vi "Main.vi"(11 "Module Admin":refnum<class "Delacor_lib_QMH_Module Admin.lvclass">) -> ()   [LabVIEW 2020, in "Acquisition .lvlib"]
doc: "This template is based off of the Queued Message Handler design pattern and the Queued Message Handler project template that ships with LabVIEW.\n\nThe main difference is that the queue is private to this module and communication between modules is performed via Broadcast and Request events.\n\nRequest events are wrapped in public API methods and are handled in the Event Handling Loop (EHL) of this VI. Any module can register for Broadcast events sent by this module. The EHL generates messages based on user interface actions.\n\nThe Message Handling Loop (MHL) processes messages generated by the EHL, or by other messages. The messages are string values, so new messages can be added easily to the Message Cases case structure in the MHL. Each message cluster can also provide an optional value for Message Data, which is a variant that can be converted to whatever message-specific data is required.\n_____\nBased on Delacor QMH Project Template 6.0.0.89."
uses:
  Acquisition .lvlib
  <vilib>/Delacor/Delacor QMH/Libraries/Module Admin_class/Delacor_lib_QMH_Module Admin.lvclass
  Module Data--cluster.ctl
  Stop Argument--cluster.ctl
  <vilib>/Delacor/Delacor QMH/Libraries/Message Queue_class/Delacor_lib_QMH_Message Queue.lvclass/Delacor_lib_QMH_Message Queue.ctl
  <vilib>/Delacor/Delacor QMH/Libraries/Module Admin_class/Delacor_lib_QMH_Module Admin.lvclass/Delacor_lib_QMH_Module Admin.ctl
  Start Analog AQ Argument--cluster.ctl
  Start Digital AQ Argument--cluster.ctl
  Stop AQ Argument--cluster.ctl
  <vilib>/Utility/miscctls.llb/LVPointTypeDef.ctl
  <vilib>/DAQmx/read.llb/DAQmx Read (Digital 1D U8 NChan 1Samp).vi
  <vilib>/DAQmx/read.llb/DAQmx Read (Analog 1D Wfm NChan NSamp).vi
  <vilib>/Delacor/Delacor QMH/Libraries/Message Queue_class/Delacor_lib_QMH_Enqueue Message (Single).vi
  <vilib>/Delacor/Delacor QMH/Libraries/Module Admin_class/Delacor_lib_QMH_Get External Launch.vi
  <vilib>/DAQmx/miscellaneous.llb/DAQmx Fill In Error Info.vi
  <vilib>/Utility/error.llb/Error Cluster From Error Code.vi
  <vilib>/ErrorRing/Error Ring.xnode
  <vilib>/Delacor/Delacor QMH/Libraries/Message Queue_class/Delacor_lib_QMH_Message Queue.lvclass
panel:
  out "error out":errorcluster
  out "Status":string
types:
  T1 = typedef "Acquisition .lvlib/Request Events--cluster.ctl" = cluster{"Stop Module":refnum<user-event>, "Show Panel":refnum<user-event>, "Hide Panel":refnum<user-event>, "Get Module Execution Status":refnum<user-event>, "Show Diagram":refnum<user-event>, "WakeUp Analog HL":refnum<user-event>, "WakeUp Digital HL":refnum<user-event>, "Put HL to Sleep":refnum<user-event>, "Start Analog AQ":refnum<user-event>, "Start Digital AQ":refnum<user-event>, "Stop AQ":refnum<user-event>}
  T2 = typedef "Acquisition .lvlib/Module Data--cluster.ctl" = cluster{"Status":string, "Analog Signal":cluster{"DAQ Board Name":tag, "Canales":tag[], "rate":dbl, "number of samples ":i32, "Tiempo":dbl}, "digital Signal":cluster{"DAQ Board Name":tag, "Canales":tag[], "rate":i32, "Tiempo ":dbl}}
  T3 = enum32{"invalid lock state", "Not Locked", "Locked (No Password)", "Password-protected"}
  T4 = typedef "Acquisition .lvlib/Stop Argument--cluster.ctl" = cluster{"Origin":string, "Exit via Stop Module Req?":bool, "Wait for Module to stop?":bool}
  T5 = typedef "Acquisition .lvlib/Start Analog AQ Argument--cluster.ctl" = cluster{"Boolean":bool}
  T6 = typedef "Acquisition .lvlib/Start Digital AQ Argument--cluster.ctl" = cluster{"Boolean":bool}
  T7 = typedef "Acquisition .lvlib/Stop AQ Argument--cluster.ctl" = cluster{"Boolean":bool}
  T8 = typedef "LVPointTypeDef.ctl" = cluster{"Horizontal":i16, "Vertical":i16}
  T9 = enum32{"Invalid", "Standard", "Closed", "Hidden", "Minimized", "Maximized"}
  T10 = cluster{"DAQ Board Name":tag, "Canales":tag[], "rate":dbl, "number of samples ":i32, "Tiempo":dbl}
  T11 = cluster{"DAQ Board Name":tag, "Canales":tag[], "rate":i32, "Tiempo ":dbl}
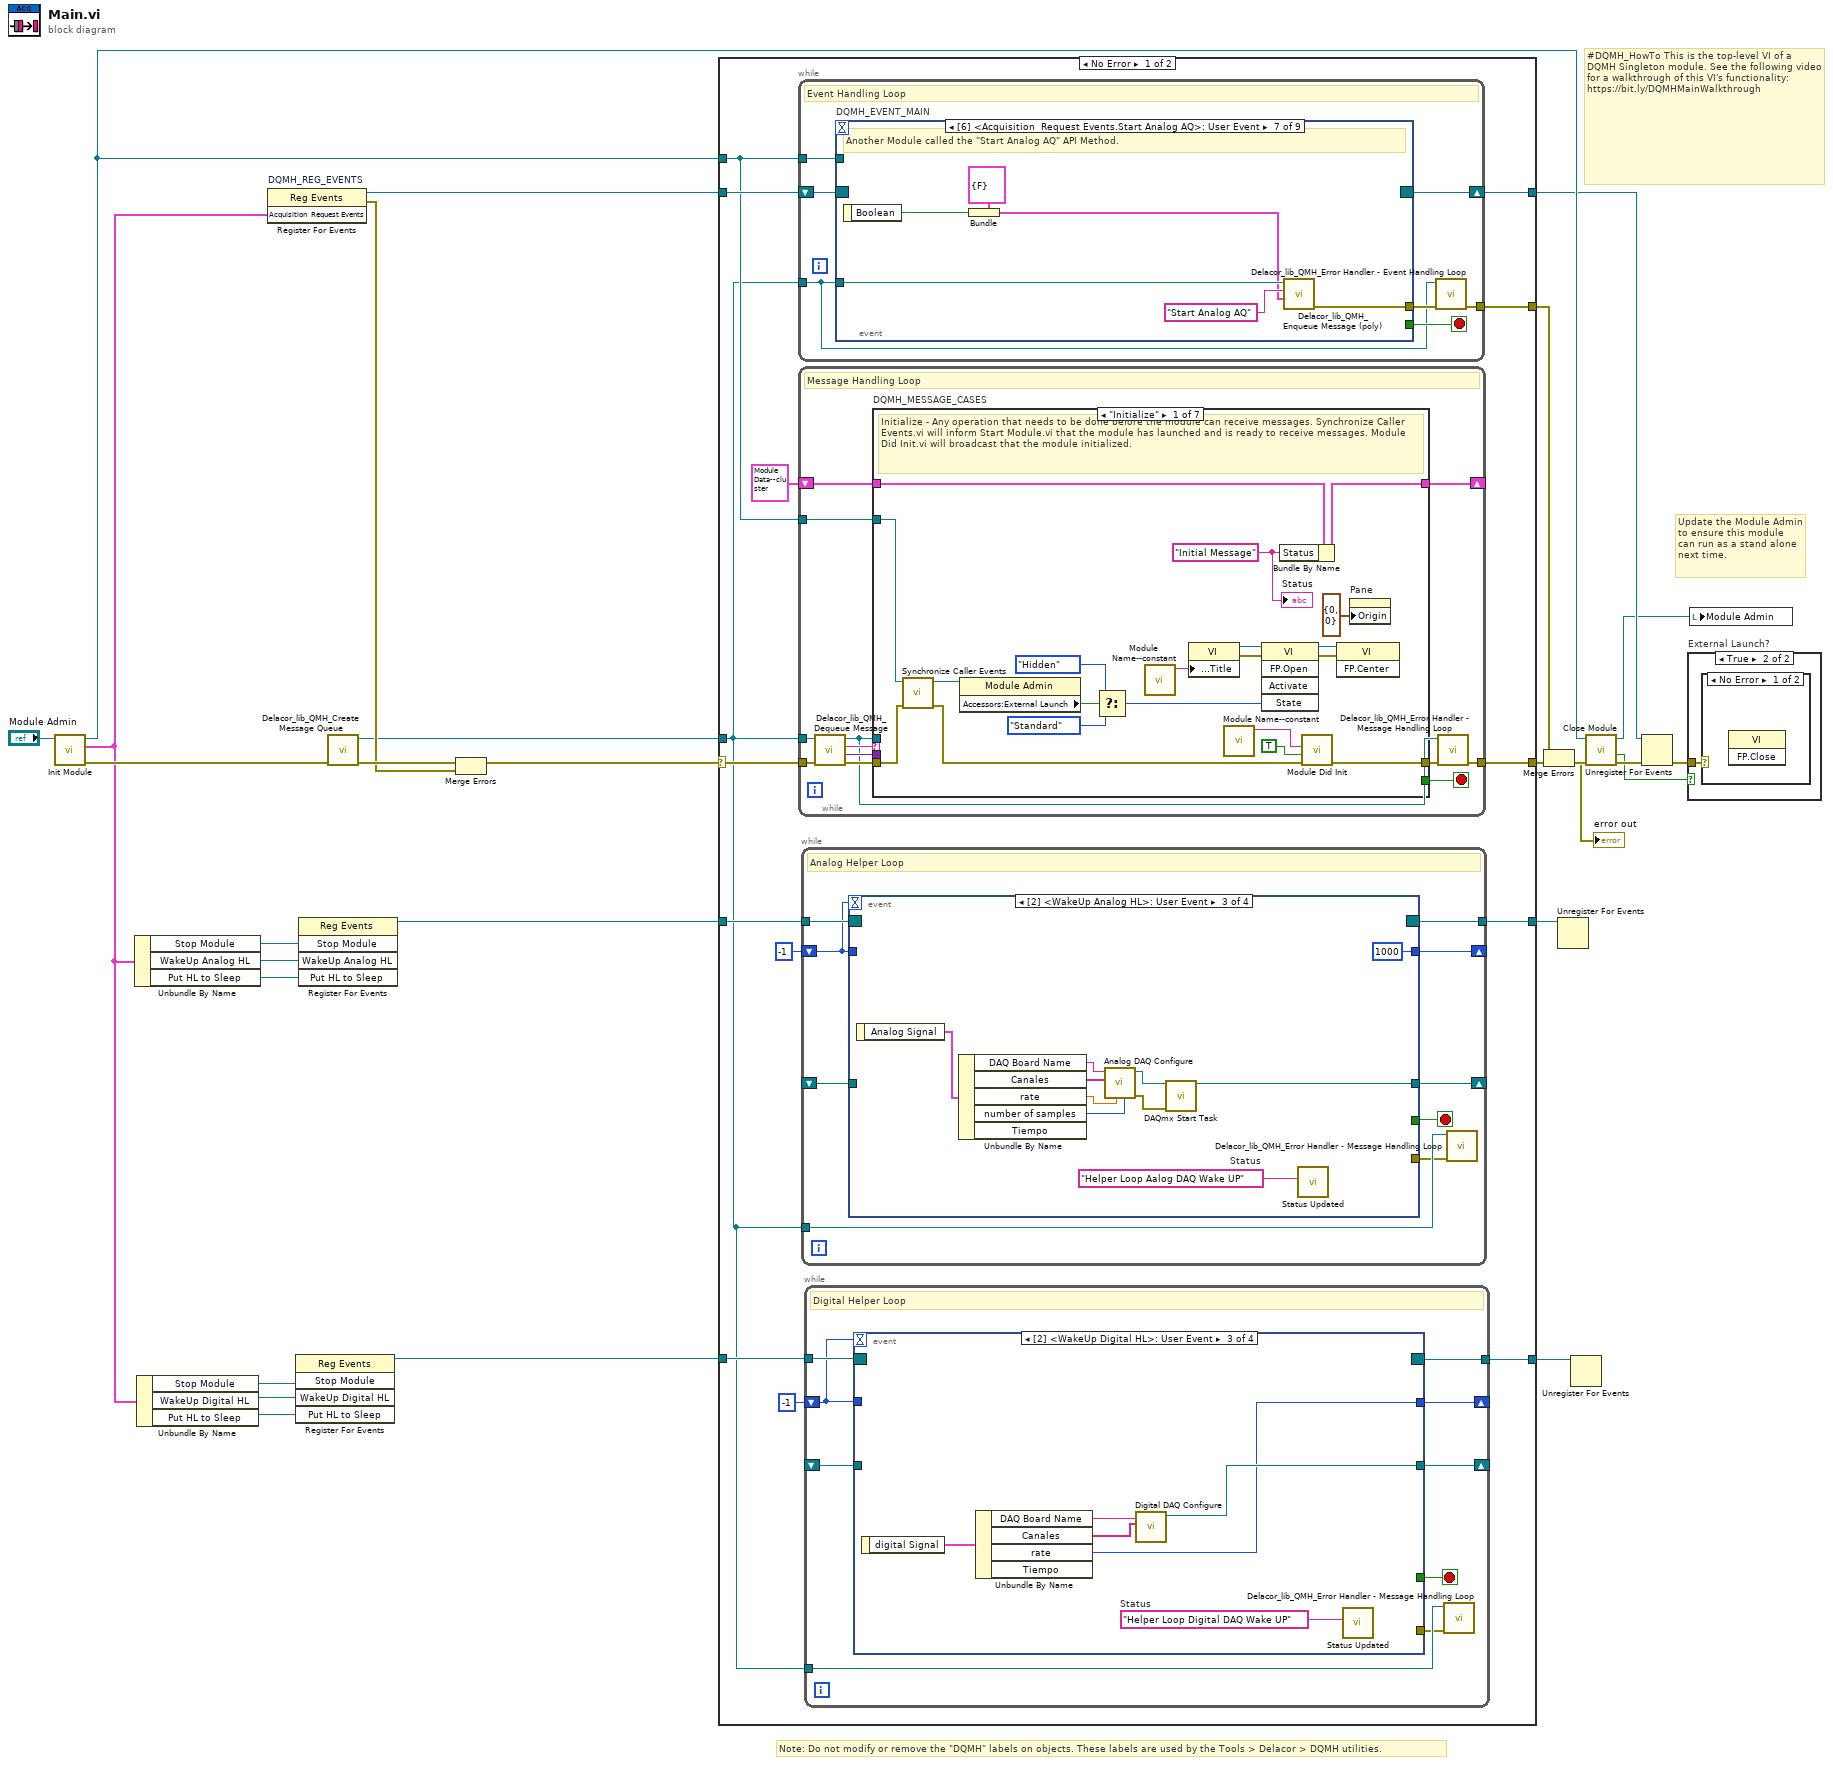
[diagram p0: block diagram]
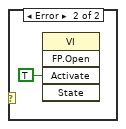
[diagram p3: hidden frame]
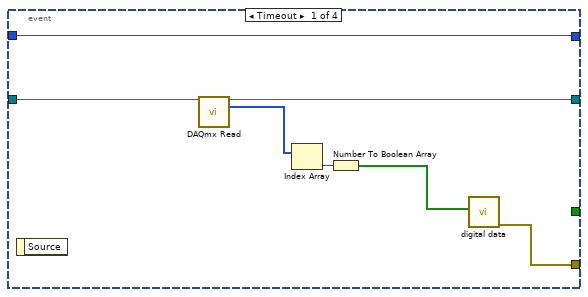
[diagram p4: hidden frame]
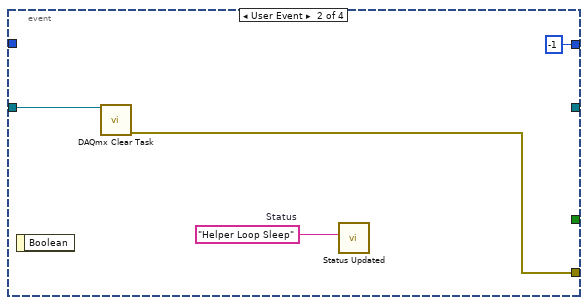
[diagram p5: hidden frame]
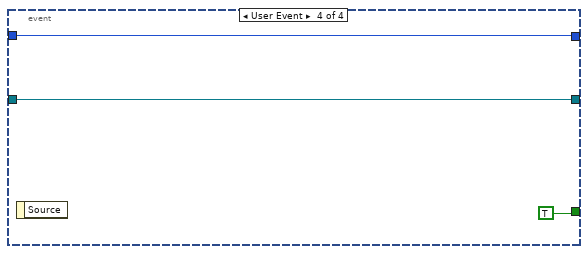
[diagram p6: hidden frame]
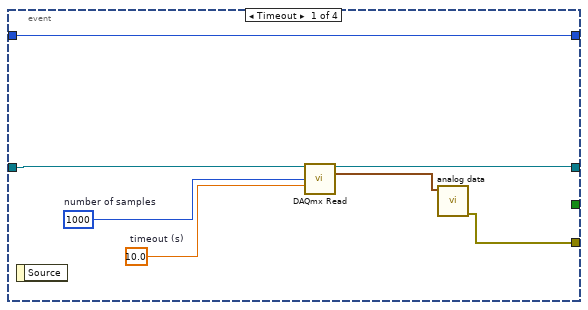
[diagram p7: hidden frame]
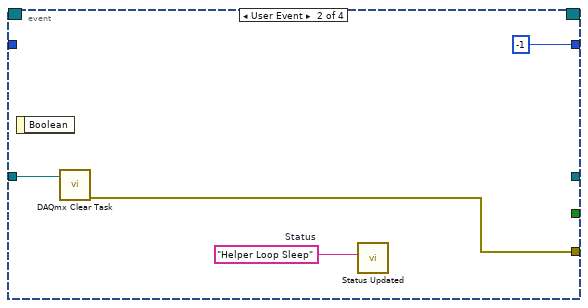
[diagram p8: hidden frame]
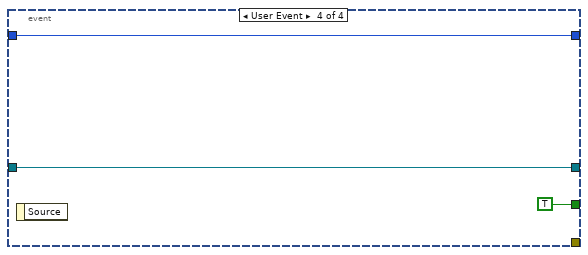
[diagram p9: hidden frame]
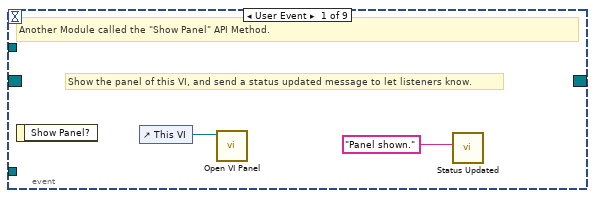
[diagram p10: hidden frame]
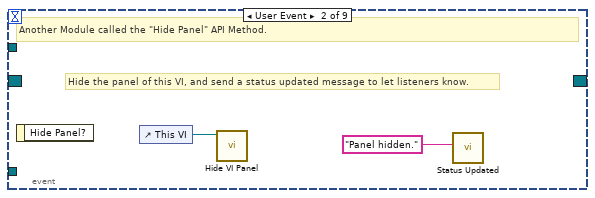
[diagram p11: hidden frame]
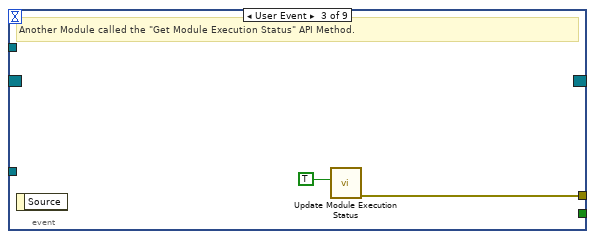
[diagram p12: hidden frame]
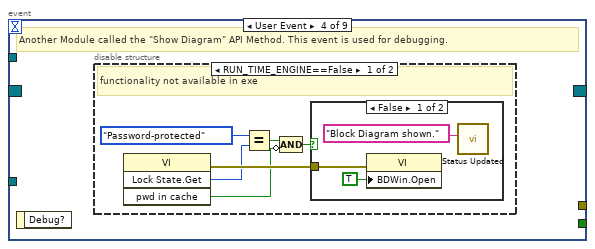
[diagram p13: hidden frame]
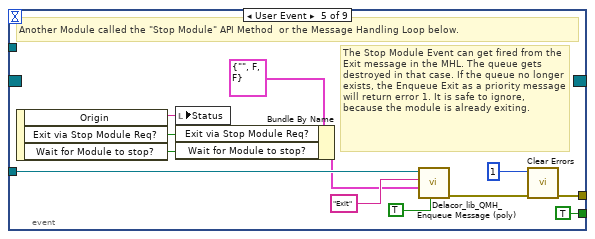
[diagram p16: hidden frame]
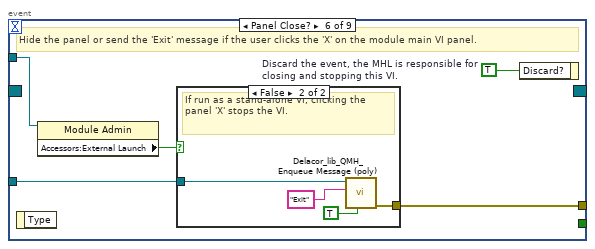
[diagram p17: hidden frame]
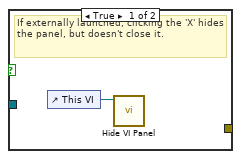
[diagram p18: hidden frame]
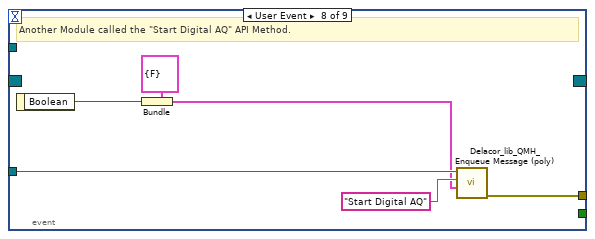
[diagram p19: hidden frame]
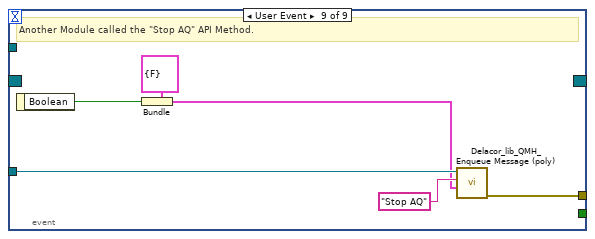
[diagram p20: hidden frame]
diagram:
  # "#DQMH_HowTo This is the top-level VI of a DQMH Singleton module. See the following video for a walkthrough of this VI's functionality: https://bit.ly/DQMHMainWalkthrough"
  # "Note: Do not modify or remove the \"DQMH\" labels on objects. These labels are used by the Tools > Delacor > DQMH utilities."
  # "Update the Module Admin to ensure this module can run as a stand alone next time."
  n1 = call "Init Module.vi"("Singleton Module Admin in"="Module Admin") -> ("error out"=w26:errorcluster, "Acquisition  Request Events"=w8:T1, "Singleton Module Admin out"=w18:refnum<class "Delacor_lib_QMH_Module Admin.lvclass">)  [unwired: 8 in]
  n2 = Unbundle By Name(w8) -> ("Stop Module"=w9:refnum<user-event>, "WakeUp Analog HL"=w10:refnum<user-event>, "Put HL to Sleep"=w11:refnum<user-event>)
  n3 = Unbundle By Name(w8) -> ("Stop Module"=w5:refnum<user-event>, "WakeUp Digital HL"=w6:refnum<user-event>, "Put HL to Sleep"=w7:refnum<user-event>)
  n4 = register-events "DQMH_REG_EVENTS"(w8) -> (reference out=w16:refnum<event-registration>, error out=w19:errorcluster)  [unwired: 2 in]
  n5 = register-events(w5, w6, w7) -> (reference out=w4:refnum<event-registration>)  [unwired: 2 in, 1 out]
  n6 = register-events(w9, w10, w11) -> (reference out=w3:refnum<event-registration>)  [unwired: 2 in, 1 out]
  n7 = call <vilib>:"Delacor_lib_QMH_Create Message Queue.vi"("error in"=w26) -> ("error out"=w21:errorcluster, "Message Queue"=w15:refnum<class "Delacor_lib_QMH_Message Queue.lvclass">)  [unwired: 9 in]
  n8 = Merge Errors(w21, w19) -> (w20:errorcluster)
  n9 = case shown="No Error" w20 {
    selector: w20 -> [w39 w273]
    tunnel: [w41 w272] -> w27
    tunnel: [w38 w278] -> w17
    tunnel: w16 -> [w36 w278]
    tunnel: w15 -> [w30 w271]
    tunnel: [w40 _] -> w24
    tunnel: w18 -> [w35 w274]
    tunnel: w4 -> [w34 w270]
    tunnel: w3 -> [w33 w269]
    tunnel: [w32 w270] -> w2
    tunnel: [w31 w269] -> w1
    frame No Error {
      n10 = while {
        tunnel: w30 -> [w104]
        shift-right: [w107] -> w38
        shift-left: w36 -> [w108]
        tunnel: [w109] -> w40
        tunnel: w35 -> [w105]
        stop <- w106 stop-if-true
        # "Event Handling Loop"
        n11 = event "DQMH_EVENT_MAIN" shown="[6] <Acquisition  Request Events.Start Analog AQ>: User Event" {
          selector: w108 -> [_ _ _ _ _ _ _ _ _]
          dyn-events: [_ _ _ _ _ _ _ _ _] -> w107
          timeout: _ -> [_ _ _ _ _ _ _ _ _]
          tunnel: [_ _ _ _ TRUE ("Discard?") _ _ _ _] -> w106
          tunnel: w104 -> [_ _ _ _ w133 w140 w153 w159 w165]
          tunnel: [_ _ w116 _ w136 w142 w148 w154 w160] -> w110
          tunnel: w105 -> [_ _ _ _ _ w139 _ _ _]
          event User Event {
            # "Show the panel of this VI, and send a status updated message to let listeners know."
            # "Another Module called the \"Show Panel\" API Method."
            n12 = event-data() -> ()  [unwired: 1 in, 1 out]
            n13 = control-ref of="This VI"() -> (w112:refnum<vi>)
            n14 = call "Open VI Panel.vi"("VI"=w112) -> ()  [unwired: 10 in, 1 out]
            n15 = call "Status Updated.vi"("Status"="Panel shown." ("format string")) -> ()  [unwired: 10 in, 1 out]
          }
          event User Event {
            # "Hide the panel of this VI, and send a status updated message to let listeners know."
            # "Another Module called the \"Hide Panel\" API Method."
            n16 = event-data() -> ()  [unwired: 1 in, 1 out]
            n17 = control-ref of="This VI"() -> (w114:refnum<vi>)
            n18 = call "Hide VI Panel.vi"("VI"=w114) -> ()  [unwired: 10 in, 1 out]
            n19 = call "Status Updated.vi"("Status"="Panel hidden." ("format string")) -> ()  [unwired: 10 in, 1 out]
          }
          event User Event {
            # "Another Module called the \"Get Module Execution Status\" API Method."
            n20 = event-data() -> ()  [unwired: 1 in, 1 out]
            n21 = call "Update Module Execution Status.vi"("Running?"=TRUE) -> ("error out"=w116:errorcluster)  [unwired: 10 in]
          }
          event User Event {
            # "Another Module called the \"Show Diagram\" API Method. This event is used for debugging."
            n22 = event-data() -> ()  [unwired: 1 in, 1 out]
            n23 = disable-structure shown="RUN_TIME_ENGINE==False" {
              frame condition #0 (active) {
                # "functionality not available in exe"
                n24 = invoke class="VI" method="Lock State.Get"() -> (error out=w122:errorcluster, "Get Lock State"=w121:T3, "pwd in cache"=w118:bool)  [unwired: 4 in, 1 out]
                n25 = Equal?(x=T3."Password-protected", y=w121) -> (x = y?=w119:bool)
                n26 = Compound Arithmetic op=AND(w119, invert w118) -> (w117:bool)
                n27 = case shown="False" w117 {
                  tunnel: w122 -> [w125 _]
                  frame False {
                    n28 = property class="VI"(error in=w125, "BDWin.Open"=TRUE ("Block Diagram Window:Open")) -> ()  [unwired: 1 in, 2 out]
                    n29 = call "Status Updated.vi"("Status"="Block Diagram shown." ("format string")) -> ()  [unwired: 10 in, 1 out]
                  }
                  frame True {
                    # "Password-protected VI, and the password is not in the cache. Do not show the diagram."
                  }
                }
              }
              frame condition #1 {
              }
            }
          }
          event User Event {
            # "The Stop Module Event can get fired from the Exit message in the MHL. The queue gets destroyed in that case. If the queue no longer exists, the Enqueue Exit as a priority message will return error 1. It is safe to ignore, because the module is already exiting."
            # "Another Module called the \"Stop Module\" API Method  or the Message Handling Loop below."
            n30 = event-data() -> ("Origin"=w132:string, "Exit via Stop Module Req?"=w128:bool, "Wait for Module to stop?"=w127:bool)  [unwired: 1 in]
            n31 = local write "Status"(w132) -> ()
            n32 = Bundle By Name(cluster=T4 {"Origin"="", "Exit via Stop Module Req?"=FALSE, "Wait for Module to stop?"=FALSE} ("Stop Argument"), "Exit via Stop Module Req?"=w128, "Wait for Module to stop?"=w127) -> (w126:T4)
            n33 = call-poly <vilib>:"Delacor_lib_QMH_Enqueue Message (poly).vi"("Priority Message? (F)"=TRUE, "Message Data"=w126, "Message"="Exit", "Message Queue in"=w133) -> ("error out"=w137:errorcluster)  [unwired: 6 in, 1 out]
            n34 = call <vilib>:"Clear Errors.vi"("error in (no error)"=w137, "specific error code to clear (0: all)"=1) -> ("error out"=w136:errorcluster)  [unwired: 4 in, 1 out]
          }
          event Panel Close? {
            w141 = TRUE  # Discard the event, the MHL is responsible for closing and stopping this VI.
            # "Hide the panel or send the 'Exit' message if the user clicks the 'X' on the module main VI panel."
            n35 = event-data() -> ()  [unwired: 1 in, 1 out]
            n36 = property class="Module Admin"(reference=w139) -> ("Accessors:External Launch"=w138:bool)  [unwired: 1 in, 2 out]
            n37 = case shown="False" w138 {
              tunnel: w140 -> [_ w146]
              tunnel: [_ w147] -> w142
              frame True {
                # "If externally launched, clicking the 'X' hides the panel, but doesn't close it."
                n38 = control-ref of="This VI"() -> (w143:refnum<vi>)
                n39 = call "Hide VI Panel.vi"("VI"=w143) -> ()  [unwired: 10 in, 1 out]
              }
              frame False {
                # "If run as a stand-alone VI, clicking the panel 'X' stops the VI."
                n40 = call-poly <vilib>:"Delacor_lib_QMH_Enqueue Message (poly).vi"("Priority Message? (F)"=TRUE, "Message"="Exit", "Message Queue in"=w146) -> ("error out"=w147:errorcluster)  [unwired: 7 in, 1 out]
              }
            }
            n41 = event-data("Discard?"=w141) -> ()  [unwired: 1 in, 1 out]
          }
          event User Event {
            # "Another Module called the \"Start Analog AQ\" API Method."
            n42 = event-data() -> ("Boolean"=w149:bool)  [unwired: 1 in]
            n43 = Bundle(cluster=T5 {"Boolean"=FALSE} ("Start Analog AQ Argument"), "Boolean"=w149) -> (w150:T5)
            n44 = call-poly <vilib>:"Delacor_lib_QMH_Enqueue Message (poly).vi"("Message Data"=w150, "Message"="Start Analog AQ", "Message Queue in"=w153) -> ("error out"=w148:errorcluster)  [unwired: 7 in, 1 out]
          }
          event User Event {
            # "Another Module called the \"Start Digital AQ\" API Method."
            n45 = event-data() -> ("Boolean"=w155:bool)  [unwired: 1 in]
            n46 = Bundle(cluster=T6 {"Boolean"=FALSE} ("Start Digital AQ Argument"), "Boolean"=w155) -> (w156:T6)
            n47 = call-poly <vilib>:"Delacor_lib_QMH_Enqueue Message (poly).vi"("Message Data"=w156, "Message"="Start Digital AQ", "Message Queue in"=w159) -> ("error out"=w154:errorcluster)  [unwired: 7 in, 1 out]
          }
          event User Event {
            # "Another Module called the \"Stop AQ\" API Method."
            n48 = event-data() -> ("Boolean"=w161:bool)  [unwired: 1 in]
            n49 = Bundle(cluster=T7 {"Boolean"=FALSE} ("Stop AQ Argument"), "Boolean"=w161) -> (w162:T7)
            n50 = call-poly <vilib>:"Delacor_lib_QMH_Enqueue Message (poly).vi"("Message Data"=w162, "Message"="Stop AQ", "Message Queue in"=w165) -> ("error out"=w160:errorcluster)  [unwired: 7 in, 1 out]
          }
        }
        n51 = call-dynamic "Delacor_lib_QMH_Error Handler - Event Handling Loop.vi"("error in"=w110, "Message Queue in"=w104) -> ("dup error in"=w109:errorcluster)  [unwired: 8 in, 1 out]
      }
      n52 = while {
        tunnel: w30 -> [w168]
        shift-right: [w172] -> _
        shift-left: T2 {"Status"="", "Analog Signal"={"DAQ Board Name"="", "Canales"=[], "rate"=0.0, "number of samples "=0, "Tiempo"=0.0}, "digital Signal"={"DAQ Board Name"="", "Canales"=[], "rate"=1000, "Tiempo "=1000.0}} ("Data Cluster") -> [w173]
        tunnel: w39 -> [w176]
        tunnel: [w174] -> w41
        tunnel: w35 -> [w166]
        stop <- w171 stop-if-true
        # "Message Handling Loop"
        n53 = call-dynamic "Delacor_lib_QMH_Dequeue Message.vi"("error in"=w176, "Message Queue in"=w168) -> ("error out"=w175:errorcluster, "Message Data"=w169:variant, "Message"=w170:string, "Message Queue out"=w167:refnum<class "Delacor_lib_QMH_Message Queue.lvclass">)  [unwired: 6 in]
        n54 = case "DQMH_MESSAGE_CASES" shown="\"Initialize\"" w170 {
          selector: w170 -> [_ _ _ w230 _ _ _]
          tunnel: w167 -> [_ w200 w222 _ _ _ _]
          tunnel: w175 -> [w195 w207 w228 w232 w251 w260 w268]
          tunnel: [w193 w203 w225 w233 w245 w254 w262] -> w177
          tunnel: w173 -> [w184 w202 w221 w231 w246 w255 w267]
          tunnel: [w183 w202 w221 w231 w246 w255 w267] -> w172
          tunnel: [_ _ w220 _ _ _ _] -> w171
          tunnel: w169 -> [_ w201 w219 _ w249 w258 w265]
          tunnel: w166 -> [w185 w199 w214 _ _ _ _]
          frame "Initialize" {
            w179 = "Initial Message" ("Initial Message")
            # "Initialize - Any operation that needs to be done before the module can receive messages. Synchronize Caller Events.vi will inform Start Module.vi that the module has launched and is ready to receive messages. Module Did Init.vi will broadcast that the module initialized."
            n55 = call "Synchronize Caller Events.vi"("error in (no error)"=w195, "Singleton Module Admin in"=w185) -> ("error out"=w194:errorcluster, "Singleton Module Admin out"=w180:refnum<class "Delacor_lib_QMH_Module Admin.lvclass">)  [unwired: 8 in]
            n56 = property class="Module Admin"(reference=w180) -> ("Accessors:External Launch"=w189:bool)  [unwired: 1 in, 2 out]
            n57 = Select(t=T9."Hidden" ("State"), s=w189, f=T9."Standard" ("State")) -> (s? t:f=w186:T9)
            n58 = call "Module Name--constant.vi"() -> ("Module Name"=w192:string)  [unwired: 11 in]
            n59 = property class="VI"("Front Panel.Title"=w192) -> (reference out=w191:refnum<vi>, error out=w197:errorcluster)  [unwired: 2 in]
            n60 = call "Module Name--constant.vi"() -> ("Module Name"=w181:string)  [unwired: 11 in]
            n61 = invoke class="VI" method="FP.Open"(reference=w191, error in=w197, "State"=w186) -> (reference out=w190:refnum<vi>, error out=w196:errorcluster)  [unwired: 2 in, 3 out]
            n62 = Bundle By Name(cluster=w184, "Status"=w179) -> (w183:T2)
            n63 = call "Module Did Init.vi"("error in (no error)"=w194, "Initialized?"=TRUE, "Origin"=w181) -> ("error out"=w193:errorcluster)  [unwired: 8 in]
            n64 = invoke class="VI" method="FP.Center"(reference=w190, error in=w196) -> ()  [unwired: 1 in, 3 out]
            n65 = property on="Pane" class="Pane"("Origin"=T8 {"Horizontal"=0, "Vertical"=0}) -> ()  [unwired: 2 in, 2 out]
            "Status" <- w179
          }
          frame "Error" {
            # "#CodeRecommended - If you ever change the name of this \"Error\" message, you'll need to update the name in the Check Loop Error.vi as well."
            # "#CodeRecommended - If the module is running in standalone mode (External Launch = FALSE), this code will pop up an error dialog and call the 'Exit' message if an error occurs. Add more fine-grained error handling here."
            # "Error - Check the error message data and respond accordingly. This message is sent by the \"Error Handler\" VIs at the end of each loop in this application."
            n66 = property class="Module Admin"(reference=w199) -> ("Accessors:External Launch"=w198:bool)  [unwired: 1 in, 2 out]
            n67 = Variant To Data(error in=w207, type=errorcluster {"status"=FALSE, "code"=0, "source"=""} ("error constant"), Variant=w201) -> (data=w208:errorcluster, error out=w205:errorcluster)
            n68 = call "Error Reported.vi"("Error"=w208) -> ()  [unwired: 10 in, 1 out]
            n69 = case shown="False" w198 {
              tunnel: [w213 _] -> w204
              tunnel: w200 -> [w211 _]
              tunnel: w208 -> [w212 _]
              frame False {
                # "If the module is running standalone, then pop up an error dialog and call the \"Exit\" message."
                n70 = call <vilib>:"Simple Error Handler.vi"("error in (no error)"=w212) -> ()  [unwired: 4 in, 5 out]
                n71 = call-poly <vilib>:"Delacor_lib_QMH_Enqueue Message (poly).vi"("Priority Message? (F)"=TRUE, "Message"="Exit", "Message Queue in"=w211) -> ("error out"=w213:errorcluster)  [unwired: 7 in, 1 out]
              }
              frame True {
                # "If the module was launched externally, calling the Error Reported broadcast VI is the only action performed by the \"Error\" message. The module's caller can then process the error appropriately."
              }
            }
            n72 = Merge Errors(w205, w204) -> (w203:errorcluster)
            n73 = local write "error out"(w203) -> ()
          }
          frame "Exit" {
            w218 = 91  # 91: not all Exit messages will have an argument
            w220 = TRUE  # Stop the VI
            # "Release the message queue reference"
            # "#CodeNeeded - Add any required cleanup code here"
            # "Exit - Exit the application."
            n74 = Variant To Data(error in=w228, type=T4 {"Origin"="", "Exit via Stop Module Req?"=FALSE, "Wait for Module to stop?"=FALSE} ("Stop Argument"), Variant=w219) -> (data=w216:T4, error out=w224:errorcluster)
            n75 = call <vilib>:"Clear Errors.vi"("error in (no error)"=w224, "specific error code to clear (0: all)"=w218) -> ("error out"=w227:errorcluster)  [unwired: 4 in, 1 out]
            n76 = control-ref of="This VI"() -> (w215:refnum<vi>)
            n77 = call-dynamic "Delacor_lib_QMH_Release Message Queue.vi"("error in"=w227, "Message Queue"=w222) -> ("error out"=w226:errorcluster)  [unwired: 9 in]
            n78 = call "Handle Exit.vi"("Stop Argument"=w216, "Admin in"=w214, "VI reference"=w215) -> ("error out"=w223:errorcluster)  [unwired: 7 in, 1 out]
            n79 = Merge Errors(w226, w223) -> (w225:errorcluster)
          }
          frame Default {
            # "'Default' case only runs if there is a message that isn't defined in any of the other cases.  Output a programming error."
            n80 = call "Module Name--constant.vi"() -> ("Module Name"=w229:string)  [unwired: 11 in]
            n81 = xnode "Error Ring"("parameter 0"=w230, "parameter 1"=w229) -> ("error out"=w234:errorcluster)
            n82 = Merge Errors(w232, w234) -> (w233:errorcluster)
          }
          frame "Start Analog AQ" {
            # "#wakeUp_analog__HL"
            # "start the analog acquisition"
            n83 = Variant To Data(error in=w251, type=T5 {"Boolean"=FALSE} ("Start Analog AQ Argument"), Variant=w249) -> (data=w247:T5, error out=w250:errorcluster)
            n84 = Unbundle By Name(w247) -> ()  [unwired: 1 out]
            n85 = Unbundle By Name(w246) -> ("Analog Signal"=w243:T10)
            n86 = call "WakeUp Analog HL.vi"("Analog Signal"=w243) -> ("error out"=w244:errorcluster)  [unwired: 10 in]
            n87 = Merge Errors(w244, w250) -> (w245:errorcluster)
          }
          frame "Start Digital AQ" {
            # "#wakeUp_digital__HL"
            # "Start to acquire digital data"
            n88 = Variant To Data(error in=w260, type=T6 {"Boolean"=FALSE} ("Start Digital AQ Argument"), Variant=w258) -> (data=w256:T6, error out=w259:errorcluster)
            n89 = Unbundle By Name(w256) -> ()  [unwired: 1 out]
            n90 = Unbundle By Name(w255) -> ("digital Signal"=w252:T11)
            n91 = call "WakeUp Digital HL.vi"("digital Signal"=w252) -> ("error out"=w253:errorcluster)  [unwired: 10 in]
            n92 = Merge Errors(w253, w259) -> (w254:errorcluster)
          }
          frame "Stop AQ" {
            # "stop to acquire data"
            n93 = Variant To Data(error in=w268, type=T7 {"Boolean"=FALSE} ("Stop AQ Argument"), Variant=w265) -> (data=w263:T7, error out=w266:errorcluster)
            n94 = Unbundle By Name(w263) -> ()  [unwired: 1 out]
            n95 = call "Put HL to Sleep.vi"() -> ("error out"=w261:errorcluster)  [unwired: 11 in]
            n96 = Merge Errors(w261, w266) -> (w262:errorcluster)
          }
        }
        n97 = call-dynamic "Delacor_lib_QMH_Error Handler - Message Handling Loop.vi"("error in"=w177, "Message Queue in"=w167) -> ("dup error in"=w174:errorcluster)  [unwired: 8 in, 1 out]
      }
      n98 = while {
        tunnel: w33 -> [w79]
        tunnel: [w77] -> w31
        tunnel: w30 -> [w76]
        shift-right: [w75] -> _
        shift-left: _ -> [w74]
        shift-right: [w73] -> _
        shift-left: -1 -> [w72]
        stop <- w78 stop-if-true
        # "Analog Helper Loop"
        n99 = event shown="[2] <WakeUp Analog HL>: User Event" {
          selector: w79 -> [_ _ _ _]
          dyn-events: [_ _ _ _] -> w77
          timeout: w72 -> [_ _ _ _]
          tunnel: [_ _ _ TRUE] -> w78
          tunnel: [w82 _ w96 w101] -> w75
          tunnel: w74 -> [w83 w89 _ w101]
          tunnel: [w86 -1 1000 w102] -> w73
          tunnel: w72 -> [w86 _ _ w102]
          tunnel: [w81 w87 _ _] -> w71
          event Timeout {
            w84 = 10.0  # timeout (s)
            w85 = 1000  # number of samples
            n100 = event-data() -> ()  [unwired: 1 in, 1 out]
            n101 = call-poly <vilib>:"DAQmx Read.vi"("task/channels in"=w83, "number of samples per channel"=w85, "timeout"=w84) -> ("task out"=w82:refnum<k21>, "data"=w80:waveform(dbl)[])  [unwired: 10 in, 1 out]
            n102 = call "analog data.vi"("data"=w80) -> ("error out"=w81:errorcluster)  [unwired: 10 in]
          }
          event User Event {
            w90 = "Helper Loop Sleep"  # Status
            n103 = event-data() -> ()  [unwired: 1 in, 1 out]
            n104 = call <vilib>:"DAQmx Clear Task.vi"("task in"=w89) -> ("error out"=w87:errorcluster)  [unwired: 14 in]
            n105 = call "Status Updated.vi"("Status"=w90) -> ()  [unwired: 10 in, 1 out]
          }
          event User Event {
            w97 = "Helper Loop Aalog DAQ Wake UP"  # Status
            n106 = event-data() -> ("Analog Signal"=w100:T10)  [unwired: 1 in]
            n107 = Unbundle By Name(w100) -> ("DAQ Board Name"=w94:tag, "Canales"=w93:tag[], "rate"=w92:dbl, "number of samples"=w91:i32)  [unwired: 1 out]
            n108 = call "Analog DAQ Configure.vi"("number of samples"=w91, "rate"=w92, "Canales"=w93, "DAQ Board Name"=w94) -> ("error out"=w99:errorcluster, "task out"=w98:refnum<k21>)  [unwired: 6 in]
            n109 = call <vilib>:"DAQmx Start Task.vi"("task/channels in"=w98, "error in"=w99) -> ("task out"=w96:refnum<k21>)  [unwired: 12 in, 1 out]
            n110 = call "Status Updated.vi"("Status"=w97) -> ()  [unwired: 10 in, 1 out]
          }
          event User Event {
            n111 = event-data() -> ()  [unwired: 1 in, 1 out]
          }
        }
        n112 = call-dynamic "Delacor_lib_QMH_Error Handler - Message Handling Loop.vi"("error in"=w71, "Message Queue in"=w76) -> ()  [unwired: 8 in, 2 out]
      }
      n113 = while {
        tunnel: w34 -> [w50]
        tunnel: [w48] -> w32
        tunnel: w30 -> [w47]
        shift-right: [w46] -> _
        shift-left: _ -> [w45]
        shift-right: [w44] -> _
        shift-left: -1 -> [w43]
        stop <- w49 stop-if-true
        # "Digital Helper Loop"
        n114 = event shown="[2] <WakeUp Digital HL>: User Event" {
          selector: w50 -> [_ _ _ _]
          dyn-events: [_ _ _ _] -> w48
          timeout: w43 -> [_ _ _ _]
          tunnel: [_ _ _ TRUE] -> w49
          tunnel: [w55 _ w66 w68] -> w46
          tunnel: w45 -> [w56 w60 _ w68]
          tunnel: [w57 -1 w64 w69] -> w44
          tunnel: w43 -> [w57 _ _ w69]
          tunnel: [w54 w59 _ _] -> w42
          event Timeout {
            n115 = event-data() -> ()  [unwired: 1 in, 1 out]
            n116 = call-poly <vilib>:"DAQmx Read.vi"("task/channels in"=w56) -> ("task out"=w55:refnum<k21>, "data"=w51:u8[])  [unwired: 12 in, 1 out]
            n117 = Index Array(array=w51) -> (element=w52:u8)  [unwired: 1 in]
            n118 = Number To Boolean Array(number=w52) -> (Boolean array=w53:bool[])
            n119 = call "digital data.vi"("Digital Signals"=w53) -> ("error out"=w54:errorcluster)  [unwired: 10 in]
          }
          event User Event {
            w58 = "Helper Loop Sleep"  # Status
            n120 = event-data() -> ()  [unwired: 1 in, 1 out]
            n121 = call <vilib>:"DAQmx Clear Task.vi"("task in"=w60) -> ("error out"=w59:errorcluster)  [unwired: 14 in]
            n122 = call "Status Updated.vi"("Status"=w58) -> ()  [unwired: 10 in, 1 out]
          }
          event User Event {
            w65 = "Helper Loop Digital DAQ Wake UP"  # Status
            n123 = event-data() -> ("digital Signal"=w67:T11)  [unwired: 1 in]
            n124 = Unbundle By Name(w67) -> ("DAQ Board Name"=w63:tag, "Canales"=w62:tag[], "rate"=w64:i32)  [unwired: 1 out]
            n125 = call "Digital DAQ Configure.vi"("Port Digitales"=w62, "DAQmx Device Digital"=w63) -> ("task out"=w66:refnum<k21>)  [unwired: 8 in, 1 out]
            n126 = call "Status Updated.vi"("Status"=w65) -> ()  [unwired: 10 in, 1 out]
          }
          event User Event {
            n127 = event-data() -> ()  [unwired: 1 in, 1 out]
          }
        }
        n128 = call-dynamic "Delacor_lib_QMH_Error Handler - Message Handling Loop.vi"("error in"=w42, "Message Queue in"=w47) -> ()  [unwired: 8 in, 2 out]
      }
    }
    frame Error {
      # "Synchronize Caller Events.vi will inform Start Module.vi that the module has launched and will let the code calling Start Module.vi register for broadcasts and would permit the caller receive the broadcast that an error occurred at launch time."
      n129 = call-dynamic "Delacor_lib_QMH_Release Message Queue.vi"("error in"=w273, "Message Queue"=w271) -> ("error out"=w272:errorcluster)  [unwired: 9 in]
      n130 = call "Synchronize Caller Events.vi"("Singleton Module Admin in"=w274) -> ("error out"=w279:errorcluster)  [unwired: 9 in, 1 out]
      n131 = call "Module Name--constant.vi"() -> ("Module Name"=w277:string)  [unwired: 11 in]
      n132 = Format Into String(format string="An error occurred during initialization. %s is no longer running.", w277) -> (resulting string=w275:string)  [unwired: 2 in, 1 out]
      n133 = Merge Errors(w272, w279) -> (w280:errorcluster)
      n134 = call "Error Reported.vi"("Additional Information"=w275, "Error"=w280) -> ()  [unwired: 9 in, 1 out]
    }
  }
  n135 = Merge Errors(w24, w27) -> (w23:errorcluster)
  n136 = Unregister For Events(event registration refnum=w1) -> ()  [unwired: 1 in, 1 out]
  n137 = Unregister For Events(event registration refnum=w2) -> ()  [unwired: 1 in, 1 out]
  n138 = call "Close Module.vi"("error in (no error)"=w23, "Module Admin in"=w18) -> ("error out"=w25:errorcluster, "External Launch"=w12:bool, "Module Admin out"=w13:refnum<class "Delacor_lib_QMH_Module Admin.lvclass">)  [unwired: 7 in]
  n139 = Unregister For Events(event registration refnum=w17, error in=w25) -> (error out=w22:errorcluster)
  "error out" <- w22
  n140 = case "External Launch?" shown="True" w12 {
    tunnel: w22 -> [_ w281]
    frame False {
    }
    frame True {
      n141 = case shown="No Error" w281 {
        frame No Error {
          n142 = invoke class="VI" method="FP.Close"() -> ()  [unwired: 3 in, 3 out]
        }
        frame Error {
          n143 = invoke class="VI" method="FP.Open"("Activate"=TRUE ("Activate?")) -> ()  [unwired: 4 in, 5 out]
        }
      }
    }
  }
  n144 = local write "Module Admin"(w13) -> ()
